vi "CopyDataToCPU.vi"(1 "Array Dst IN Host":u8[](array[numeric]), 4 "Error IN Toolkit":i32, 5 "Error IN LabVIEW":errorcluster) -> (15 "Array Dst OUT Host":u8[](array[numeric]), 18 "Error OUT Toolkit":i32, 19 "Error OUT LabVIEW":errorcluster)   [LabVIEW 2018]
doc: "It copies into a 1D U8 array stored in the CPU the results of a 1D U8 array that is stored in the GPU and it returns the array in CPU. It receives an initial 1D U8 array and an integer indicating the error.\nFor correct operation, you must pass the error that comes from VI that are using the CUDA image processing DLL"
uses:
  dll/LibreriaAutis_3.dll
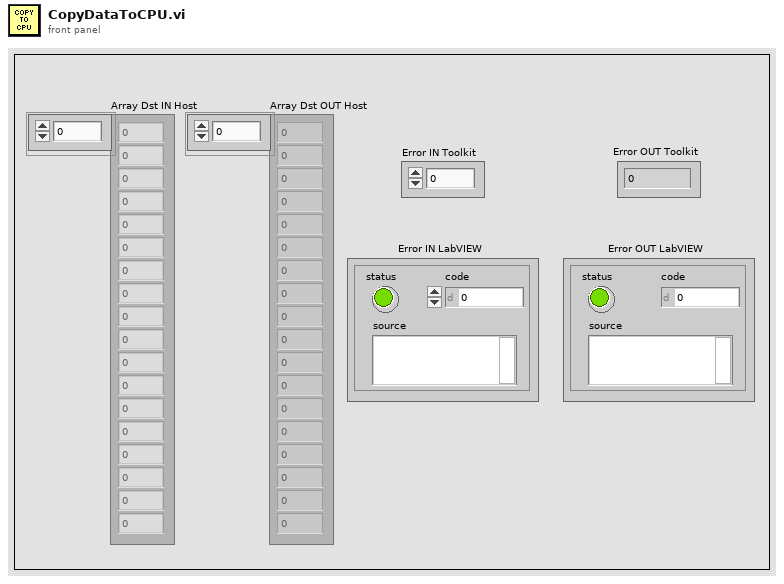
[diagram p1: front panel]
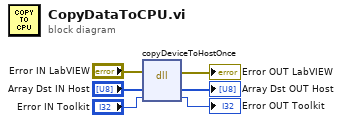
[diagram p0: block diagram]
diagram:
  n1 = dll-call lib="C:/Users/AUTIS/Desktop/LibreriaAUTIS/LabVIEW/dll/LibreriaAutis_3.dll" fn="copyDeviceToHostOnce"(error in="Error IN LabVIEW", "dst"="Array Dst IN Host", "error"="Error IN Toolkit") -> (error out=→"Error OUT LabVIEW":errorcluster, "dst"=→"Array Dst OUT Host":u8[], "error"=→"Error OUT Toolkit":i32)  [unwired: 3 in, 1 out]
